vi "PID Feedback.vi"(0 "Measured":dbl, 1 "Proportional":dbl, 2 "Integral":dbl, 3 "Derivative":dbl, 5 "Measured upper limit":dbl, 7 "Measured lower limit":dbl, 9 "Target":dbl, 11 "Feedback offset if measured exceed limits":dbl, 12 "Cycle time":dbl, 13 "Feedback low limit":dbl, 14 "Feedback high limit":dbl) -> (4 "Feedback":dbl, 15 "Error":dbl)   [LabVIEW 2018]
panel:
  out "IntegratorValue":dbl
  in  "Reset":bool
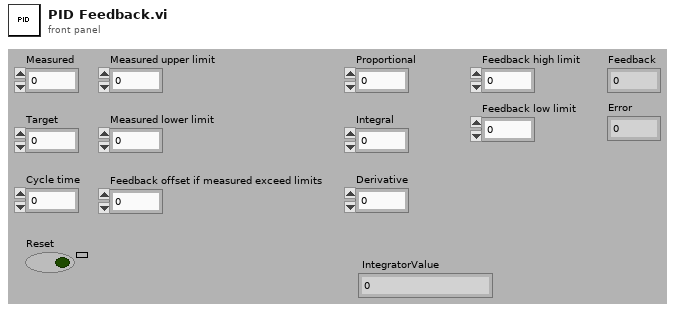
[diagram p1: front panel]
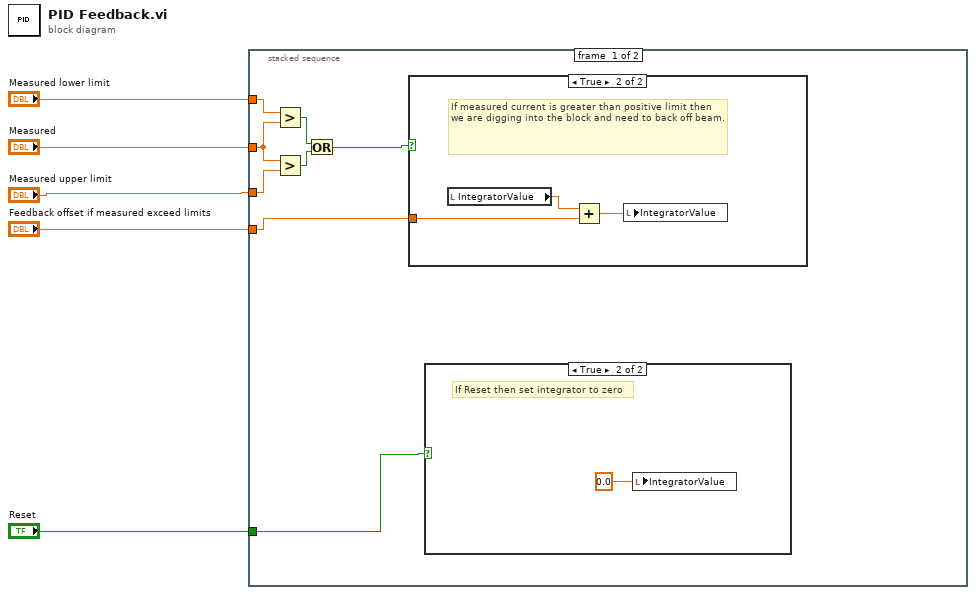
[diagram p0: block diagram]
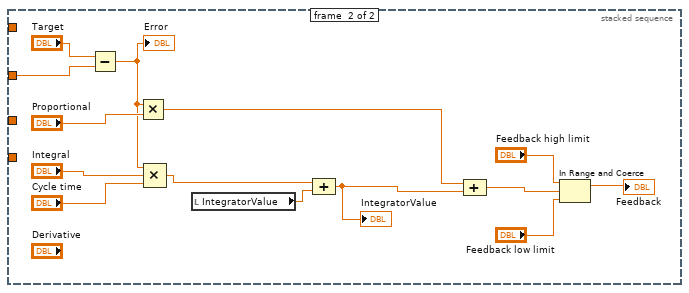
[diagram p4: hidden frame]
diagram:
  n1 = stacked-sequence {
    tunnel: "Measured" -> [w9 w20]
    tunnel: "Reset" -> [w13 _]
    tunnel: "Measured upper limit" -> [w12 _]
    tunnel: "Feedback offset if measured exceed limits" -> [w11 _]
    tunnel: "Measured lower limit" -> [w10 _]
    frame #0 {
      n2 = Greater?(x=w10, y=w9) -> (0:w6:bool)
      n3 = Greater?(x=w9, y=w12) -> (0:w8:bool)
      n4 = Or(x=w6, y=w8) -> (x .or. y?=w7:bool)
      n5 = case shown="True" w7 {
        tunnel: w11 -> [_ w14]
        frame False {
        }
        frame True {
          # "If measured current is greater than positive limit then we are digging into the block and need to back off beam."
          n6 = local read "IntegratorValue"() -> (w16:dbl)
          n7 = Add(x=w16, y=w14) -> (x+y=w15:dbl)
          n8 = local write "IntegratorValue"(w15) -> ()
        }
      }
      n9 = case shown="True" w13 {
        frame False {
        }
        frame True {
          # "If Reset then set integrator to zero"
          n10 = local write "IntegratorValue"(0.0 ("IntegratorValue")) -> ()
        }
      }
    }
    frame #1 {
      n11 = Subtract(x="Target", y=w20) -> (x-y=w29:dbl)
      "Error" <- w29
      n12 = Multiply(x=w29, y="Proportional") -> (x*y=w23:dbl)
      n13 = Compound Arithmetic op=MULTIPLY(w29, "Integral", "Cycle time") -> (w27:dbl)
      n14 = local read "IntegratorValue"() -> (w18:dbl)
      n15 = Compound Arithmetic op=ADD(w27, w18) -> (w19:dbl)
      "IntegratorValue" <- w19
      n16 = Compound Arithmetic op=ADD(w23, w19) -> (w22:dbl)
      n17 = In Range and Coerce(upper limit="Feedback high limit", x=w22, lower limit="Feedback low limit") -> (coerced(x)=→"Feedback":dbl)  [unwired: 1 out]
    }
  }
